vi "json_cache_decode.vi"(8 "error in (no error)":errorcluster, 11 "json":string) -> (0 "error out":errorcluster, 3 "cache id":u64)   [LabVIEW 2017]
uses:
  json_parse_value.vi
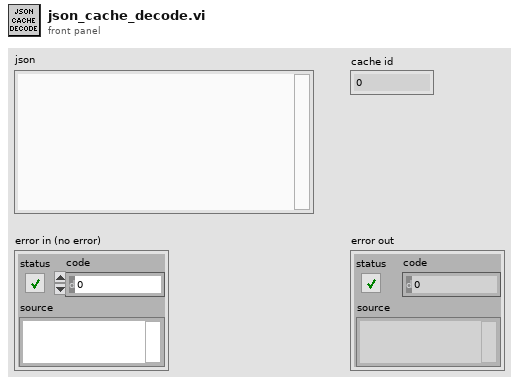
[diagram p1: front panel]
types:
  T1 = typedef "json_element.ctl" = cluster{"path":string, "type":T2, "value":variant}
  T2 = typedef "json_element_type.ctl" = enum8{"null", "bool", "int", "uint", "float", "string", "array", "object"}
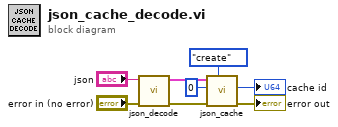
[diagram p0: block diagram]
diagram:
  n1 = call "json_decode.vi"("error in (no error)"="error in (no error)", "json"="json") -> ("error out"=w6:errorcluster, "elements"=w4:T1[])  [unwired: 8 in]
  n2 = call "json_cache.vi"("action"=enum8{"null", "get", "create", "delete"}."create", "error in (no error)"=w6, "cache id in"=u64 0 ("id in"), "elements in"=w4) -> ("error out"=→"error out":errorcluster, "cache id out"=→"cache id":u64)  [unwired: 3 in, 3 out]
